vi "Excel Protect Worksheets.vi"(0 "Sheets Ref In":refnum<k7>, 1 "Workbook Ref In":refnum<k7>, 11 "Error In":errorcluster) -> (3 "Workbook Ref Out":refnum<k7>, 4 "Sheets Ref Out":refnum<k7>, 15 "Error Out":errorcluster)   [LabVIEW 2013]
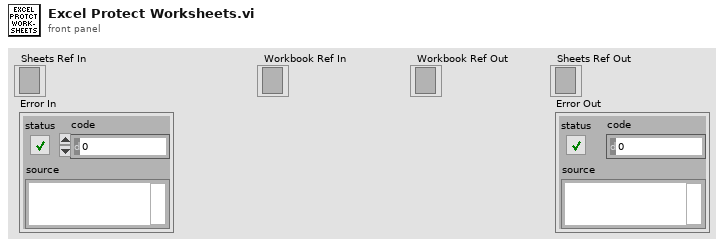
[diagram p1: front panel]
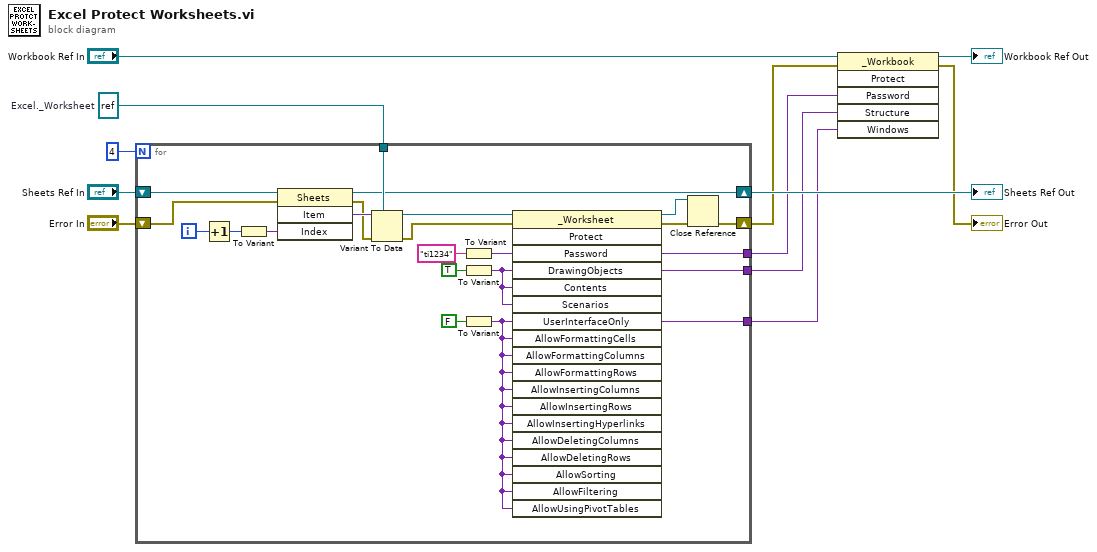
[diagram p0: block diagram]
diagram:
  w12 = refnum<k7> refnum  # Excel._Worksheet
  n1 = for {
    N: 4 -> [_]
    tunnel: w12 -> [w25]
    shift-right: [w22] -> w8
    shift-left: "Sheets Ref In" -> [w23]
    shift-right: [w17] -> w6
    shift-left: "Error In" -> [w16]
    tunnel: [w15] -> w3
    tunnel: [w14] -> w2
    tunnel: [w13] -> w1
    i -> [w21]
    n2 = Increment(x=w21) -> (x+1=w20:i32)
    n3 = To Variant(anything=w20) -> (Variant=w28:variant)
    n4 = invoke class="Sheets" method="Item"(reference=w23, error in=w16, "Index"=w28) -> (reference out=w22:refnum<k7>, error out=w27:errorcluster, "Item"=w29:variant)  [unwired: 1 in, 1 out]
    n5 = Variant To Data(error in=w27, type=w25, Variant=w29) -> (data=w26:refnum<k7>, error out=w24:errorcluster)
    n6 = To Variant(anything="ti1234") -> (Variant=w15:variant)
    n7 = To Variant(anything=TRUE) -> (Variant=w14:variant)
    n8 = To Variant(anything=FALSE) -> (Variant=w13:variant)
    n9 = invoke class="_Worksheet" method="Protect"(reference=w26, error in=w24, "Password"=w15, "DrawingObjects"=w14, "Contents"=w14, "Scenarios"=w14, "UserInterfaceOnly"=w13, "AllowFormattingCells"=w13, "AllowFormattingColumns"=w13, "AllowFormattingRows"=w13, "AllowInsertingColumns"=w13, "AllowInsertingRows"=w13, "AllowInsertingHyperlinks"=w13, "AllowDeletingColumns"=w13, "AllowDeletingRows"=w13, "AllowSorting"=w13, "AllowFiltering"=w13, "AllowUsingPivotTables"=w13) -> (reference out=w19:refnum<k7>, error out=w18:errorcluster)  [unwired: 1 in, 17 out]
    n10 = Close Reference(reference=w19, error in (no error)=w18) -> (error out=w17:errorcluster)
  }
  "Sheets Ref Out" <- w8
  n11 = invoke class="_Workbook" method="Protect"(reference="Workbook Ref In", error in=w6, "Password"=w3, "Structure"=w2, "Windows"=w1) -> (reference out=→"Workbook Ref Out":refnum<k7>, error out=→"Error Out":errorcluster)  [unwired: 1 in, 4 out]
